vi "CRYGet Text Data in Text Graph.vi"(11 "Text Graph Control Ref":refnum<vi>) -> (3 "Flatten Data String":string)   [LabVIEW 2013]
panel:
  in  "Text Format":T1
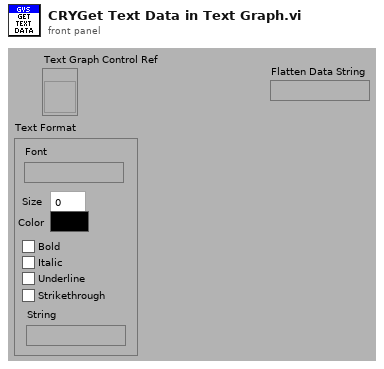
[diagram p1: front panel]
types:
  T1 = cluster{"Size":u32, "Bold":bool, "Italic":bool, "Underline":bool, "Strikethrough":bool, "Color":u32, "Font":string, "String":string}
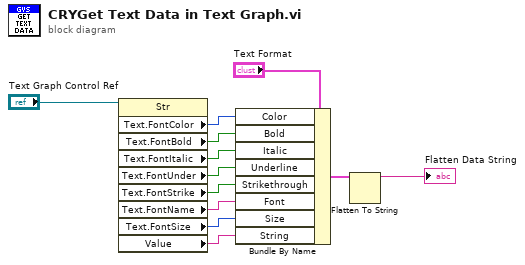
[diagram p0: block diagram]
diagram:
  n1 = property class="Str"(reference="Text Graph Control Ref") -> ("Text.FontColor"=w10:u32, "Text.FontBold"=w9:bool, "Text.FontItalic"=w8:bool, "Text.FontUnder"=w7:bool, "Text.FontStrike"=w6:bool, "Text.FontName"=w5:string, "Text.FontSize"=w4:u32, "Value"=w3:string)  [unwired: 1 in, 2 out]
  n2 = Bundle By Name(cluster="Text Format", "Color"=w10, "Bold"=w9, "Italic"=w8, "Underline"=w7, "Strikethrough"=w6, "Font"=w5, "Size"=w4, "String"=w3) -> (w2:T1)
  n3 = Flatten To String(anything=w2) -> (data string=→"Flatten Data String":string)  [unwired: 3 in, 2 out]
